vi "Create Temperature graph.vi"(8 "error in (no error)":errorcluster, 11 "Refnum in":refnum<k34>) -> (0 "error out":errorcluster, 1 "Min and Max Temperatures":dbl[][](array[numeric]), 2 "Waveform":waveform(dbl), 3 "Refnum out":refnum<k34>)   [LabVIEW 2015]
uses:
  <vilib>/measure/maresamp.llb/Resample Waveform (continuous).vi
  <vilib>/Waveform/WDTOps.llb/WDT Append Waveforms DBL.vi
  <vilib>/measure/NI_MAPro.lvlib
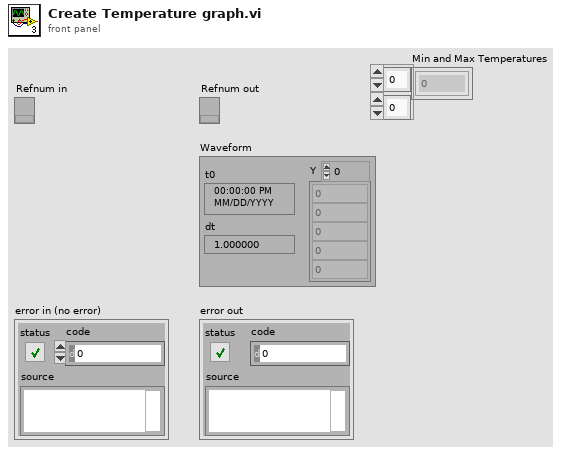
[diagram p1: front panel]
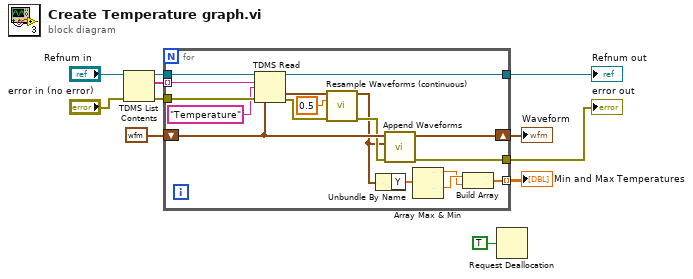
[diagram p0: block diagram]
diagram:
  n1 = TDMS List Contents(4:"error in (no error)", 7:"Refnum in") -> (0:w8:errorcluster, 2:w7:string[], 3:w6:refnum<k34>)  [unwired: 1 in, 1 out]
  n2 = for {
    tunnel: w6 -> [w28]
    tunnel: w7 -> [w27] mode=indexing
    tunnel: w8 -> [w26]
    tunnel: [w24] -> w11
    tunnel: [w21] -> w9
    shift-right: [w22] -> w3
    shift-left: waveform(dbl) {"t0"=timestamp(0 s since 1904-01-01), "dt"=0.5, "Y"=[]} ("Waveform") -> [w23]
    tunnel: [w14] -> w1 mode=indexing
    n3 = TDMS Read(0:w28, 5:w27, 7:"Temperature", 11:w26, 12:w23) -> (4:w24:refnum<k34>, 10:w17:waveform(dbl), 15:w18:errorcluster)  [unwired: 3 in, 3 out]
    n4 = call-poly <vilib>:"Resample Waveforms (continuous).vi"("waveform in"=w17, "dt"=0.5, "error in (no error)"=w18) -> ("resampled waveform out"=w15:waveform(dbl), "error out"=w16:errorcluster)  [unwired: 8 in, 3 out]
    n5 = Unbundle By Name(w15) -> ("Y"=w20:dbl[])
    n6 = call-poly <vilib>:"Append Waveforms.vi"("error in (no error)"=w16, "waveform B"=w15, "waveform A"=w23) -> ("error out"=w21:errorcluster, "waveform out"=w22:waveform(dbl))  [unwired: 7 in]
    n7 = Array Max & Min(array=w20) -> (max value=w12:dbl, min value=w13:dbl)  [unwired: 2 out]
    n8 = Build Array(w13, w12) -> (w14:dbl[])
  }
  "Refnum out" <- w11
  "Waveform" <- w3
  "error out" <- w9
  "Min and Max Temperatures" <- w1
  n9 = Request Deallocation(TRUE ("flag")) -> ()
